vi "tls handle.vi"(7 "lvlibretls connection":refnum<class "lvlibretls connection.lvclass">, 9 "server information":T3, 10 "application request in":T4, 11 "http responder in":refnum<class "https responder.lvclass">) -> (0 "connection upgrade":bool, 2 "response":T1, 3 "http responder out":refnum<class "https responder.lvclass">)   [LabVIEW 2016, in "Basic HTTPS server.lvclass"]
uses:
  Basic HTTPS server.lvclass
  HTTP responder/https responder.lvclass
  http request.ctl
  http method.ctl
  HTTP headers/http header data.ctl
  http server info.ctl
  http response.ctl
  lvlibtls/socket connection/lvlibretls connection.lvclass
  HTTP headers/http headers.lvlib
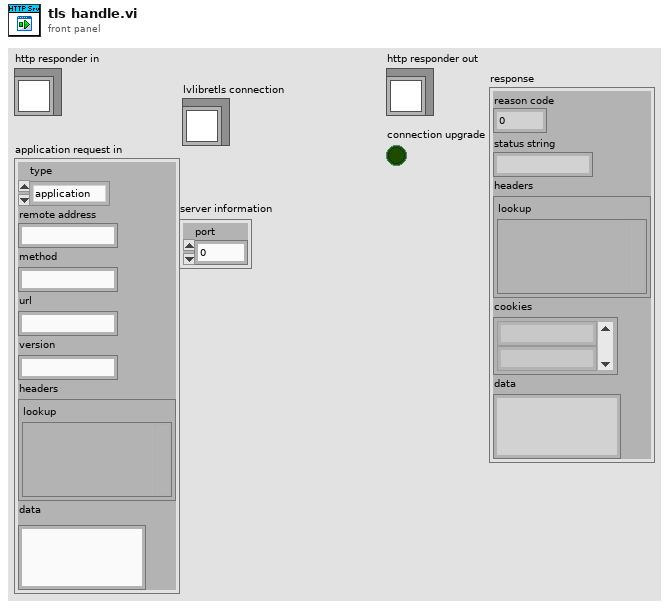
[diagram p1: front panel]
types:
  T1 = typedef "Basic HTTPS server.lvclass/http response.ctl" = cluster{"reason code":u16, "status string":string, "headers":T2, "cookies":string[], "data":string}
  T2 = typedef "http headers.lvlib/http header data.ctl" = cluster{"lookup":variant}
  T3 = typedef "Basic HTTPS server.lvclass/http server info.ctl" = cluster{"port":u16}
  T4 = typedef "Basic HTTPS server.lvclass/http request.ctl" = cluster{"type":T5, "remote address":string, "method":string, "url":string, "version":string, "headers":T2, "data":string}
  T5 = typedef "Basic HTTPS server.lvclass/http method.ctl" = enum16{"application", "error", "upgrade"}
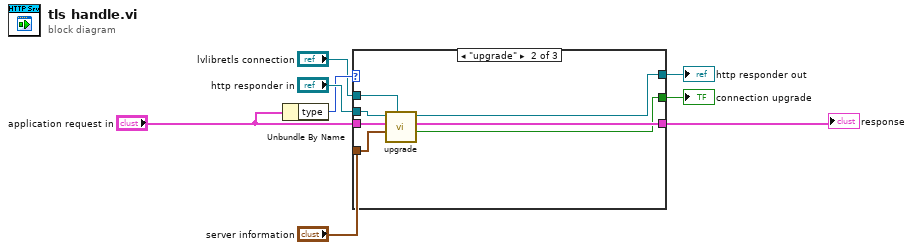
[diagram p0: block diagram]
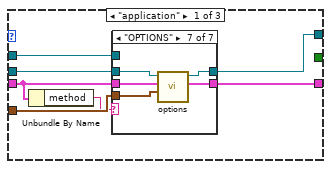
[diagram p2: hidden frame]
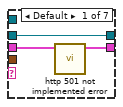
[diagram p3: hidden frame]
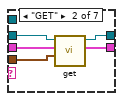
[diagram p4: hidden frame]
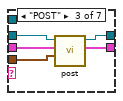
[diagram p5: hidden frame]
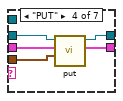
[diagram p6: hidden frame]
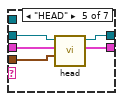
[diagram p7: hidden frame]
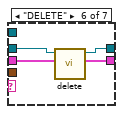
[diagram p8: hidden frame]
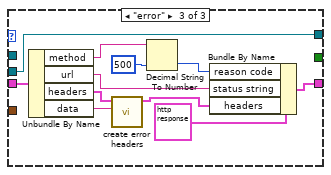
[diagram p9: hidden frame]
diagram:
  n1 = Unbundle By Name("application request in") -> ("type"=w3:T5)
  n2 = case shown="\"upgrade\"" w3 {
    tunnel: [_ w48 _] -> w8
    tunnel: "application request in" -> [w11 w54 w65]
    tunnel: "lvlibretls connection" -> [w15 w53 _]
    tunnel: "http responder in" -> [w14 w52 w64]
    tunnel: [w13 w51 w64] -> w5
    tunnel: "server information" -> [w12 w50 _]
    tunnel: [w9 w49 w55] -> w1
    frame "application" {
      n3 = Unbundle By Name(w11) -> ("method"=w10:string)
      n4 = case shown="\"OPTIONS\"" w10 {
        tunnel: w11 -> [w18 w21 w26 w31 w36 w40 w46]
        tunnel: w15 -> [_ _ _ _ _ _ _]
        tunnel: w14 -> [w17 w23 w28 w33 w38 w42 w47]
        tunnel: [w17 w22 w27 w32 w37 w41 w45] -> w13
        tunnel: w12 -> [_ w20 w25 w30 w35 _ w44]
        tunnel: [w16 w19 w24 w29 w34 w39 w43] -> w9
        frame Default {
          n5 = call "http 501 not implemented error.vi"("application request in"=w18) -> ("application request out"=w16:T1)  [unwired: 10 in]
        }
        frame "GET" {
          n6 = call-dynamic "get.vi"("server information"=w20, "application request in"=w21, "http responder in"=w23) -> ("response"=w19:T1, "http responder out"=w22:refnum<class "https responder.lvclass">)  [unwired: 7 in]
        }
        frame "POST" {
          n7 = call-dynamic "post.vi"("server information"=w25, "application request in"=w26, "http responder in"=w28) -> ("response"=w24:T1, "http responder out"=w27:refnum<class "https responder.lvclass">)  [unwired: 7 in]
        }
        frame "PUT" {
          n8 = call-dynamic "put.vi"("server information"=w30, "application request in"=w31, "http responder in"=w33) -> ("response"=w29:T1, "http responder out"=w32:refnum<class "https responder.lvclass">)  [unwired: 7 in]
        }
        frame "HEAD" {
          n9 = call-dynamic "head.vi"("server information"=w35, "application request in"=w36, "http responder in"=w38) -> ("response"=w34:T1, "http responder out"=w37:refnum<class "https responder.lvclass">)  [unwired: 7 in]
        }
        frame "DELETE" {
          n10 = call-dynamic "delete.vi"("application request in"=w40, "http responder in"=w42) -> ("response"=w39:T1, "http responder out"=w41:refnum<class "https responder.lvclass">)  [unwired: 8 in]
        }
        frame "OPTIONS" {
          n11 = call-dynamic "options.vi"("server information"=w44, "application request in"=w46, "http responder in"=w47) -> ("application response out"=w43:T1, "http responder out"=w45:refnum<class "https responder.lvclass">)  [unwired: 7 in]
        }
      }
    }
    frame "upgrade" {
      n12 = call "upgrade.vi"("lvlibretls connection"=w53, "server information"=w50, "application request in"=w54, "http responder in"=w52) -> ("upgrade successful"=w48:bool, "response"=w49:T1, "http responder out"=w51:refnum<class "https responder.lvclass">)  [unwired: 5 in]
    }
    frame "error" {
      n13 = Unbundle By Name(w65) -> ("method"=w62:string, "url"=w57:string, "headers"=w59:T2, "data"=w56:string)
      n14 = call "create error headers.vi"("custom error reason"=w56, "headers in"=w59) -> ("headers out"=w58:T2)  [unwired: 9 in]
      n15 = Decimal String To Number(string=w62, default (0L)=500 ("default (0 I32)")) -> (number=w60:i32)  [unwired: 1 in, 1 out]
      n16 = Bundle By Name(cluster=T1 {"reason code"=0, "status string"="", "headers"={"lookup"=variant}, "cookies"=[], "data"=""} ("application request"), "reason code"=w60, "status string"=w57, "headers"=w58) -> (w55:T1)
    }
  }
  "http responder out" <- w5
  "connection upgrade" <- w8
  "response" <- w1
